vi "Read Binary Configuration.vi"(7 "Type":T1, 8 "error in (no error)":errorcluster, 9 "Default If Not Found":variant, 10 "Name":string, 11 "IniFileSection in":refnum<class "IniFileSection.lvclass">) -> (0 "error out":errorcluster, 1 "Not Found?":bool, 2 "Value":variant, 3 "IniFileSection out":refnum<class "IniFileSection.lvclass">)   [LabVIEW 2019, in "IniFileSection.lvclass"]
uses:
  <vilib>/gpm_packages/@cs/Configuration/Source/IniFileSection/IniFileSection.lvclass
  <vilib>/Utility/Data Type/Type Definitions/Data Type.ctl
  <vilib>/gpm_packages/@cs/Configuration/Source/IniFileSection/IniFileSection.lvclass/IniFileSection.ctl
  <vilib>/Utility/config.llb/Read Key (String).vi
  <vilib>/Utility/config.llb/NI_LVConfig.lvlib
  <vilib>/Utility/Data Type/NI_Data Type.lvlib
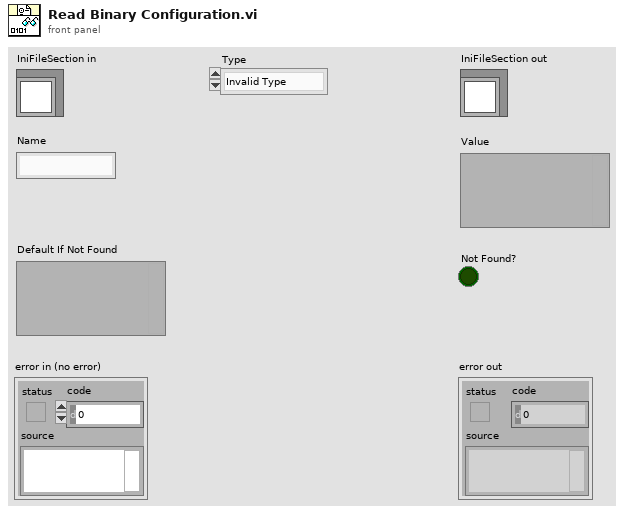
[diagram p1: front panel]
types:
  T1 = typedef "NI_Data Type.lvlib/Data Type.ctl" = enum8{"Invalid Type", "Void", "I8", "I16", "I32", "I64", "U8", "U16", "U32", "U64", "Single Float", "Double Float", "Extended Float", "Single Complex", "Double Complex", "Extended Complex", "Enum U8", "Enum U16", "Enum U32", "Enum U64", "Single Float With Unit", "Double Float With Unit", "Extended Float With Unit", "Single Complex with Unit", "Double Complex with Unit", "Extended Complex with Unit", "Boolean", "String", "Path", "Picture", "Tag", "Array", "Cluster", "Variant", "LV Variant", "Waveform", "Timestamp", "Digital Waveform", "Digital Data", "ExpressData", "Refnum", "External Data", "VI", "Poly VI", "LabVIEW Class Instance", "Fixed Point", "Set Collection", "Map Collection"}
  T2 = typedef "NI_LVConfig.lvlib/Config Data RefNum.ctl" = refnum<k1>
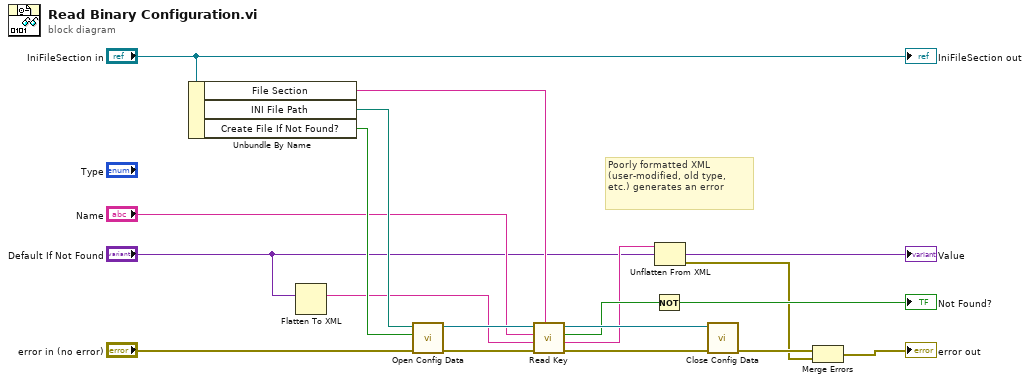
[diagram p0: block diagram]
diagram:
  # "Poorly formatted XML\n(user-modified, old type,\netc.) generates an error"
  n1 = Unbundle By Name("IniFileSection in") -> ("File Section"=w13:string, "INI File Path"=w14:path, "Create File If Not Found?"=w12:bool)
  n2 = Flatten To XML(anything="Default If Not Found") -> (xml string=w6:string)
  n3 = call <vilib>:"Open Config Data.vi"("error in (no error)"="error in (no error)", "create file if necessary (T)"=w12, "configuration file path"=w14) -> ("error out"=w19:errorcluster, "refnum"=w17:T2)  [unwired: 6 in, 1 out]
  n4 = call-poly <vilib>:"Read Key.vi"("section"=w13, "error in (no error)"=w19, "default value"=w6, "key"="Name", "refnum"=w17) -> ("error out"=w18:errorcluster, "value"=w5:string, "found?"=w15:bool, "refnum out"=w16:T2)  [unwired: 3 in]
  n5 = Not(x=w15) -> (.not. x?=→"Not Found?":bool)
  n6 = Unflatten From XML(xml string=w5, type="Default If Not Found") -> (value=→"Value":variant, error out=w2:errorcluster)  [unwired: 1 in]
  n7 = call <vilib>:"Close Config Data.vi"("error in (no error)"=w18, "refnum"=w16) -> ("error out"=w10:errorcluster)  [unwired: 8 in, 1 out]
  n8 = Merge Errors(w10, w2) -> (→"error out":errorcluster)
  "IniFileSection out" <- "IniFileSection in"
